vi "Generate Data Clusters.vi"(8 "error in (no error)":errorcluster, 11 "Item Ref in":T1 format="%.0x") -> (0 "error out":errorcluster, 1 "Outputs":T9 {"Holding Registers"."Mapping"."VS Reference" format="%.0x"; "Coils"."Mapping"."VS Reference" format="%.0x"}, 2 "Inputs":T10 {"Input Registers"."Mapping"."VS Reference" format="%.0x"; "Discrete Inputs"."Mapping"."VS Reference" format="%.0x"}, 3 "Parent Ref out":T1 format="%.0x", 4 "Input References":T8 {"Input Registers" format="%.0x"; "Discrete Inputs" format="%.0x"})   [LabVIEW 2021]
uses:
  Modbus Type.ctl
  Shared/Modbus Master Shared.lvlib
  <vilib>/NI VeriStand/Custom Device API/Custom Device Item Ref.ctl
  <vilib>/NI VeriStand/Custom Device API/Custom Device API.lvlib
  Shared/Controls/Data Model/Channel.ctl
  Shared/Controls/Data Model/Input Channel Data.ctl
  Shared/Controls/Data Model/Output Channel Data.ctl
  Shared/Controls/Data Model/Input References.ctl
  Shared/Controls/Data Model/Output References.ctl
  Shared/Controls/Data Model/DataType.ctl
  Shared/Controls/Data Model/Mapping.ctl
  <vilib>/NI VeriStand/Custom Device API/Custom Device Channel Type.ctl
panel:
  in  "Start Index":i32
  out "Channel Registers":T1[](array[typedef]) format="%.0x"
  out "End Index":i32
  out "Channels":T2[](array[typedef]) {"Mapping"."VS Reference" format="%.0x"}
  in  "Type":T3
  out "Output References":T7 {"Holding Registers" format="%.0x"; "Coils" format="%.0x"}
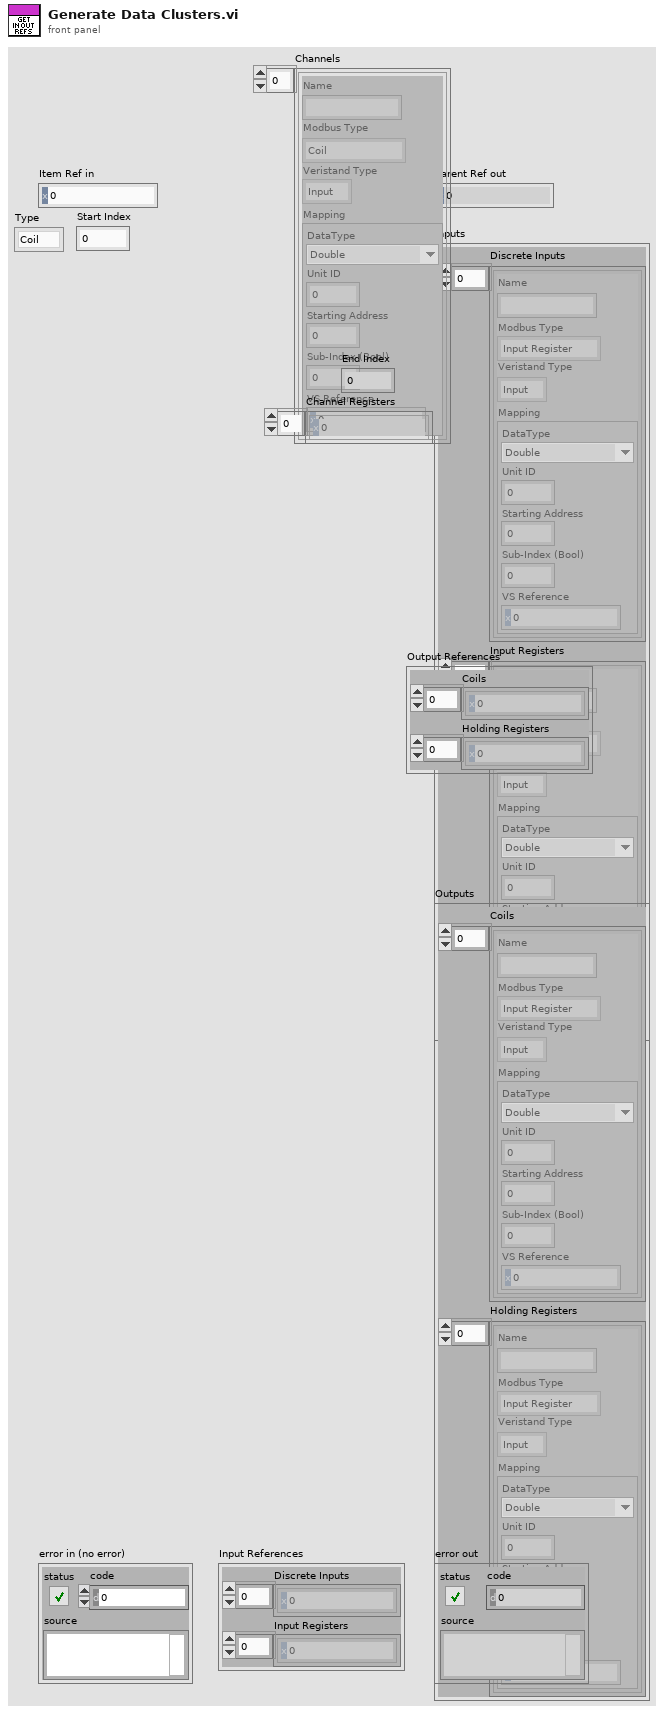
[diagram p1: front panel]
types:
  T1 = typedef "Custom Device API.lvlib/Custom Device Item Ref.ctl" = u64
  T2 = typedef "Modbus Master Shared.lvlib/Channel.ctl" = cluster{"Name":string, "Modbus Type":T3, "Veristand Type":T4, "Mapping":T5}
  T3 = typedef "Modbus Master Shared.lvlib/Modbus Type.ctl" = enum16{"Coil", "Discrete Input", "Holding Register", "Input Register"}
  T4 = typedef "Custom Device API.lvlib/Custom Device Channel Type.ctl" = enum16{"Input", "Output"}
  T5 = typedef "Modbus Master Shared.lvlib/Mapping.ctl" = cluster{"DataType":T6, "Unit ID":u8, "Starting Address":u16, "Sub-Index (Bool)":u16, "VS Reference":T1}
  T6 = typedef "Modbus Master Shared.lvlib/DataType.ctl" = enum16{"Double", "Single", "I64", "I32", "I16", "I8", "U64", "U32", "U16", "U8", "Boolean"}
  T7 = typedef "Modbus Master Shared.lvlib/Output References.ctl" = cluster{"Coils":T1[], "Holding Registers":T1[]}
  T8 = typedef "Modbus Master Shared.lvlib/Input References.ctl" = cluster{"Discrete Inputs":T1[], "Input Registers":T1[]}
  T9 = typedef "Modbus Master Shared.lvlib/Output Channel Data.ctl" = cluster{"Coils":T2[], "Holding Registers":T2[]}
  T10 = typedef "Modbus Master Shared.lvlib/Input Channel Data.ctl" = cluster{"Discrete Inputs":T2[], "Input Registers":T2[]}
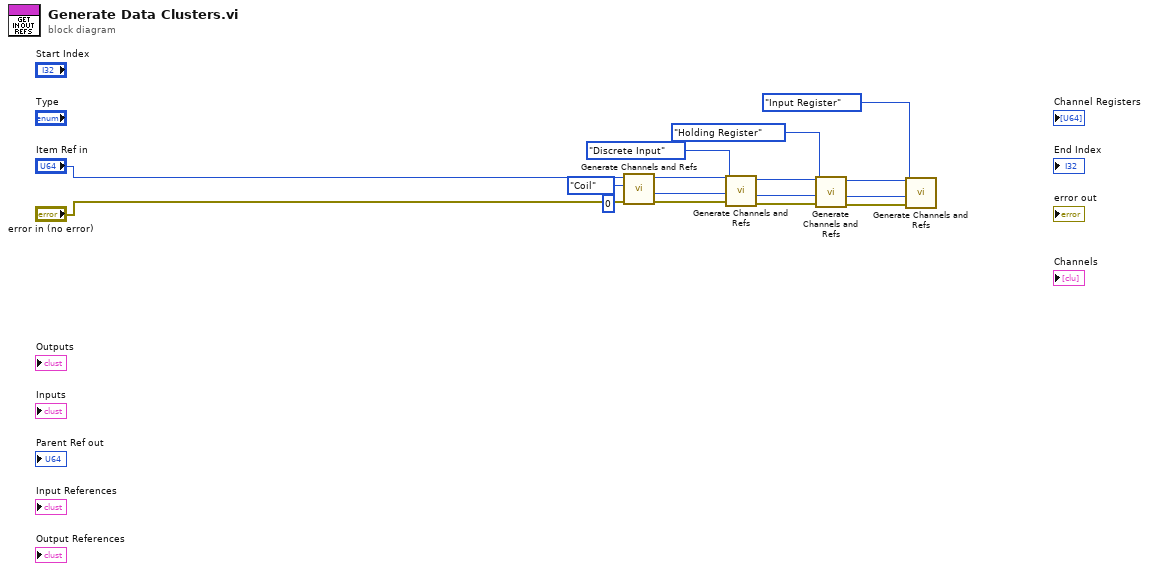
[diagram p0: block diagram]
diagram:
  n1 = call "Generate Channels and Refs.vi"("error in (no error)"="error in (no error)", "Start Index in"=0, "Type"=Modbus_Type."Coil", "Item Ref in"="Item Ref in") -> ("error out"=w5:errorcluster, "Next Index"=w12:i32, "Item Ref out"=w7:T1)  [unwired: 3 in, 2 out]
  n2 = call "Generate Channels and Refs.vi"("error in (no error)"=w5, "Start Index in"=w12, "Type"=Modbus_Type."Discrete Input", "Item Ref in"=w7) -> ("error out"=w9:errorcluster, "Next Index"=w6:i32, "Item Ref out"=w10:T1)  [unwired: 3 in, 2 out]
  n3 = call "Generate Channels and Refs.vi"("error in (no error)"=w9, "Start Index in"=w6, "Type"=Modbus_Type."Holding Register", "Item Ref in"=w10) -> ("error out"=w4:errorcluster, "Next Index"=w3:i32, "Item Ref out"=w2:T1)  [unwired: 3 in, 2 out]
  n4 = call "Generate Channels and Refs.vi"("error in (no error)"=w4, "Start Index in"=w3, "Type"=Modbus_Type."Input Register", "Item Ref in"=w2) -> ()  [unwired: 3 in, 5 out]
